vi "image_to_2d.vi"() -> ()   [LabVIEW 2015]
panel:
  out "Array":u8[][](array[numeric])
  out "24-bit pixmap":u32[][](array[numeric]) format="%x"
  in  "Path 2":path
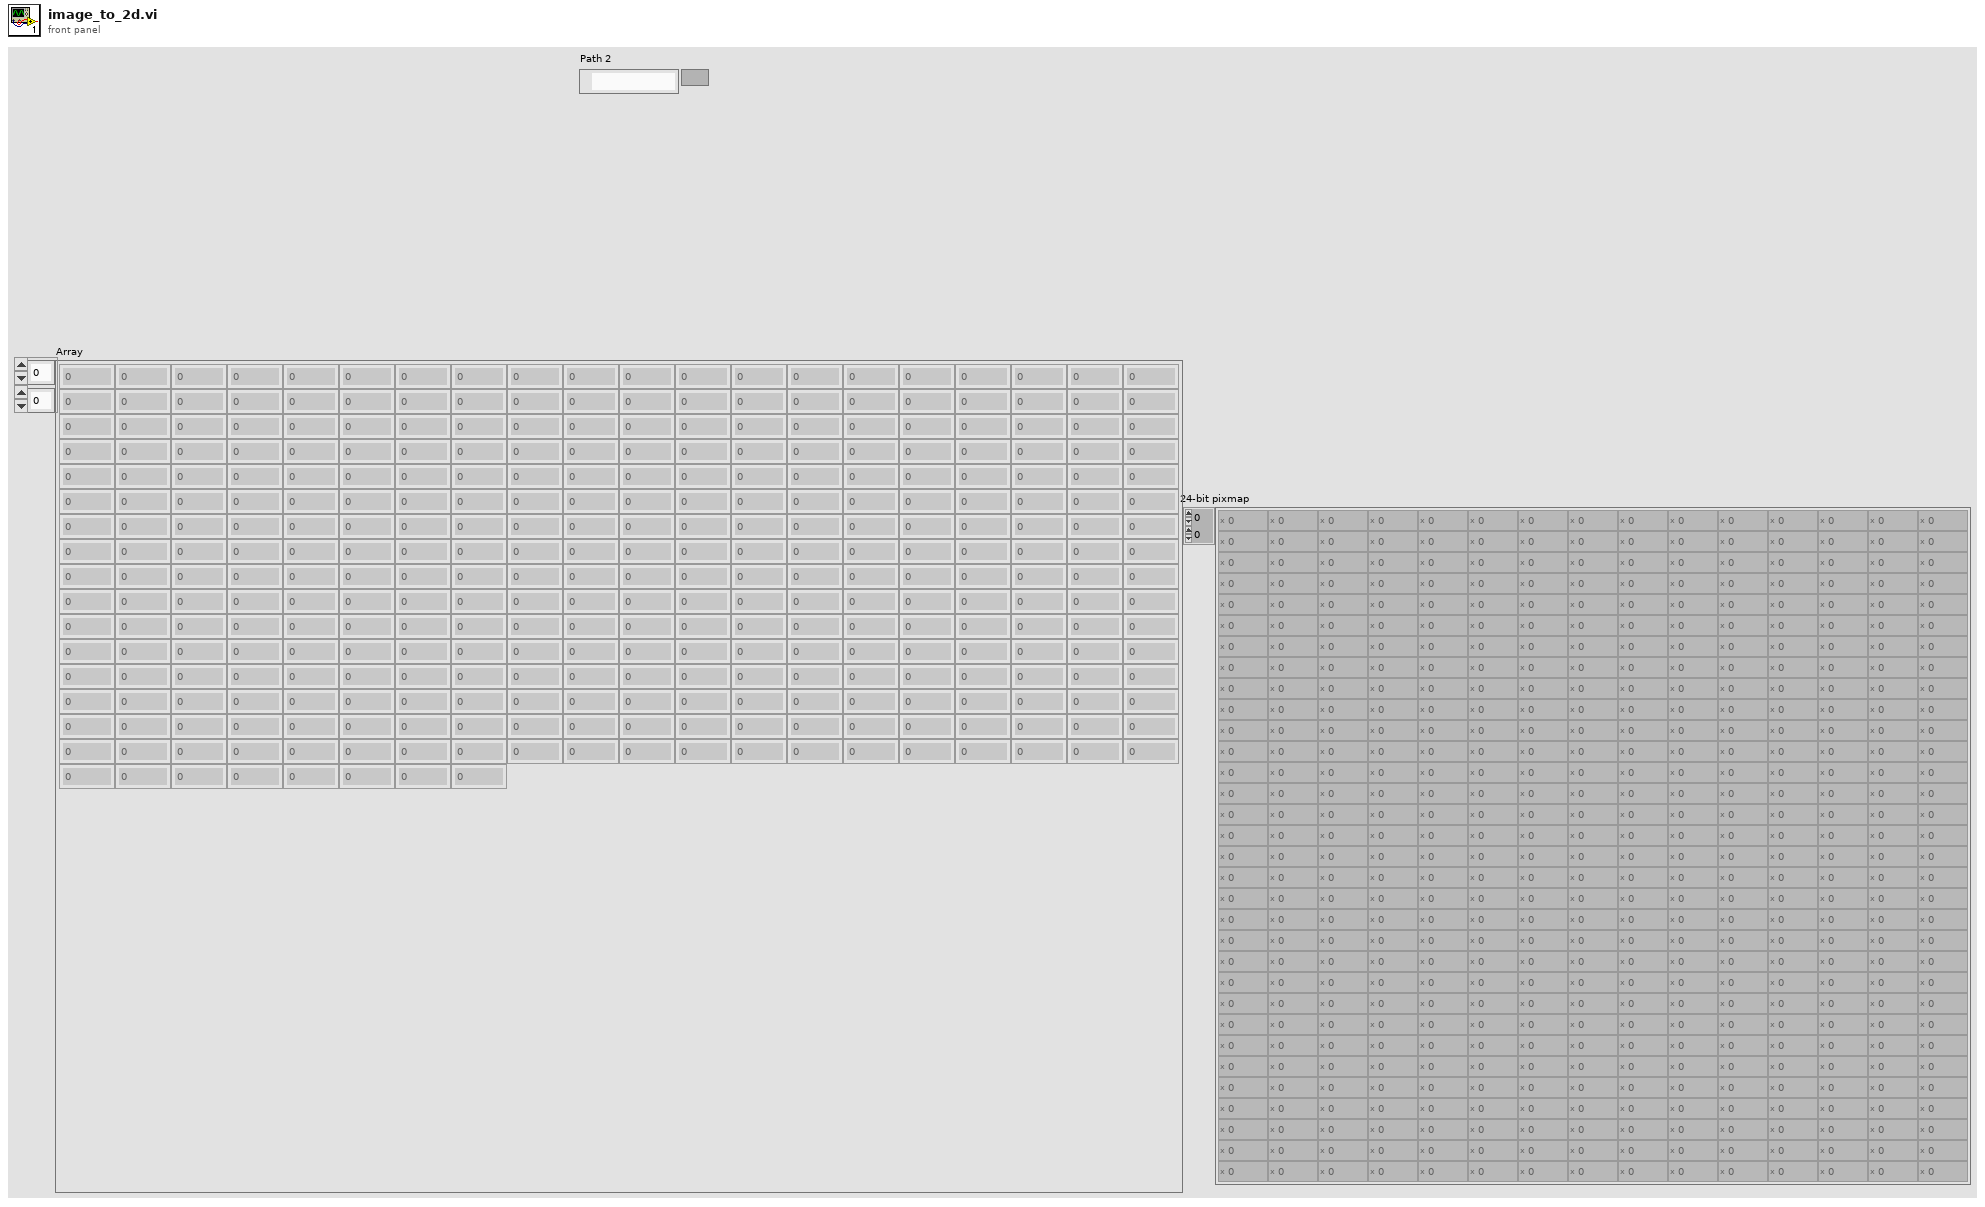
[diagram p1: front panel]
types:
  T1 = typedef "imagedata.ctl" = cluster{"image type":i32, "image depth":i32, "image":u8[], "mask":u8[], "colors":u32[], "Rectangle":cluster{"left":i16, "top":i16, "right":i16, "bottom":i16}}
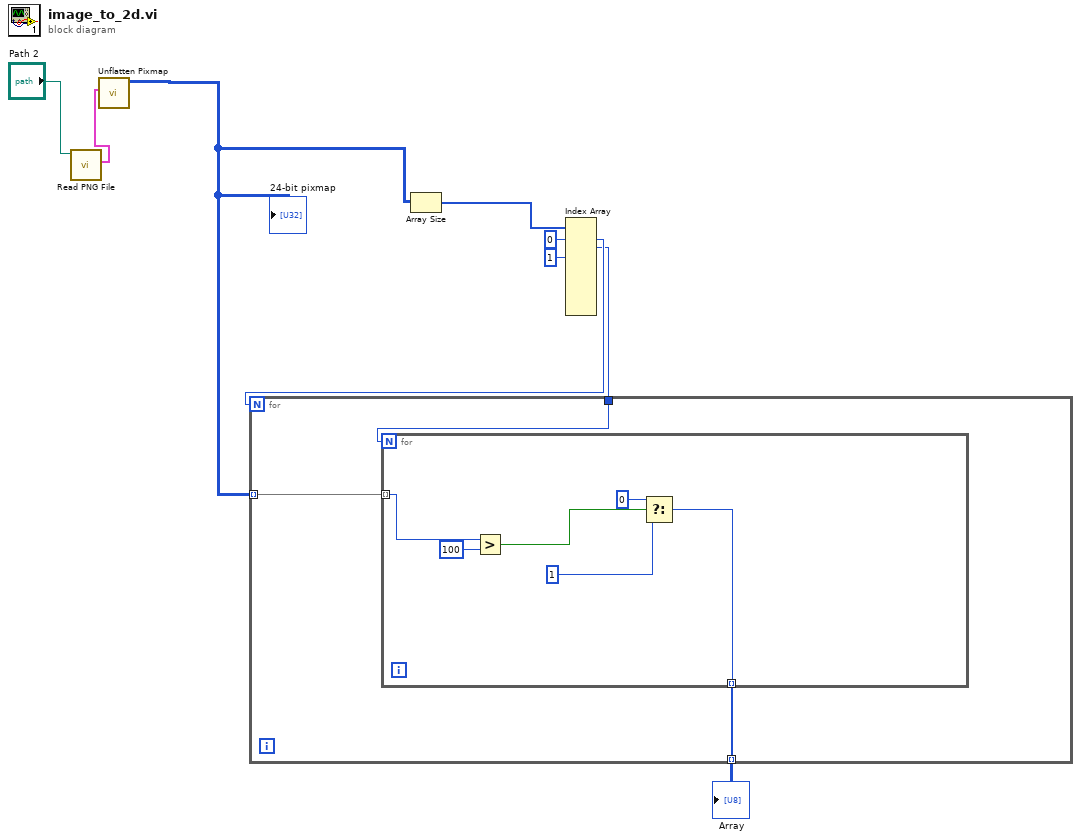
[diagram p0: block diagram]
diagram:
  n1 = call <vilib>:"Read PNG File.vi"("path to PNG file"="Path 2") -> ("image data"=w8:T1)  [unwired: 8 in, 2 out]
  n2 = call <vilib>:"Unflatten Pixmap.vi"("image data"=w8) -> ("24-bit pixmap"=w6:u32[][])  [unwired: 4 in, 6 out]
  "24-bit pixmap" <- w6
  n3 = Array Size(array=w6) -> (size(s)=w5:i32[])
  n4 = Index Array(array=w5, index #1=0 ("index"), index #2=1 ("index")) -> (element #1=w2:i32, element #2=w1:i32)  [unwired: 8 in, 8 out]
  n5 = for {
    N: w2 -> [_]
    tunnel: w6 -> [w12] mode=indexing
    tunnel: [w11] -> w7 mode=indexing
    tunnel: w1 -> [w10]
    n6 = for {
      N: w10 -> [_]
      tunnel: w12 -> [w18] mode=indexing
      tunnel: [w14] -> w11 mode=indexing
      n7 = Greater?(x=w18, y=u32 100) -> (0:w16:bool)
      n8 = Select(t=u8 0, s=w16, f=u8 1) -> (s? t:f=w14:u8)
    }
  }
  "Array" <- w7
